vi "Configure Tag Math.vi"(0 "VISA resource name":refnum<visa-resource-name>, 5 "Math Channel (001)":string="001", 7 "Tag Name (\"\")":string, 9 "Tag Number (\"\")":string, 11 "error in (no error)":errorcluster) -> (4 "VISA resource name out":refnum<visa-resource-name>, 6 "Math Channel":string, 15 "error out":errorcluster)   [LabVIEW 2020, in "Yokogawa GX Series.lvlib"]
doc: "Sets the tag of math channel.\n\nCommand: STagMath"
uses:
  <instrlib>/Yokogawa GX Series/Yokogawa GX Series.lvlib
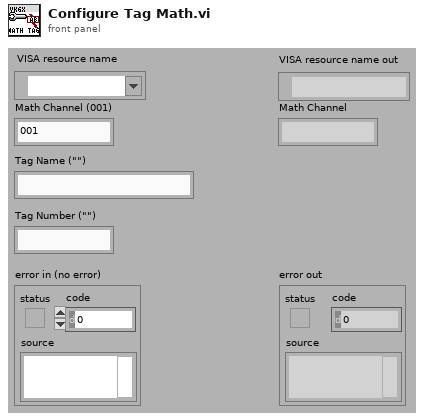
[diagram p1: front panel]
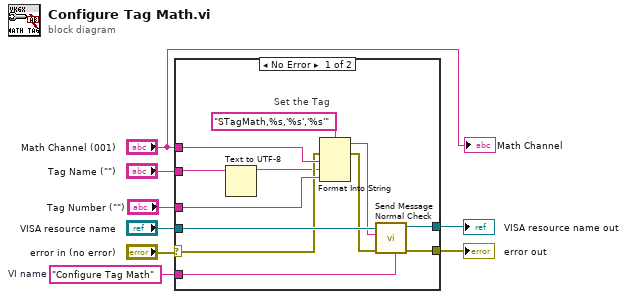
[diagram p0: block diagram]
diagram:
  w6 = "Configure Tag Math"  # VI name
  n1 = case shown="No Error" "error in (no error)" {
    selector: "error in (no error)" -> [w11 w21]
    tunnel: "Tag Name (\"\")" -> [w9 _]
    tunnel: "VISA resource name" -> [w19 w22]
    tunnel: w6 -> [w16 _]
    tunnel: [w15 w22] -> w5
    tunnel: [w14 w21] -> w4
    tunnel: "Tag Number (\"\")" -> [w13 _]
    tunnel: "Math Channel (001)" -> [w12 _]
    frame No Error {
      # "Set the Tag"
      n2 = Text to UTF-8(11:w9) -> (3:w10:string)  [unwired: 2 in, 1 out]
      n3 = Format Into String(format string="STagMath,%s,'%s','%s'", error in=w11, w12, w10, w13) -> (resulting string=w18:string, error out=w17:errorcluster)  [unwired: 1 in]
      n4 = call <instrlib>:"Send Message Normal Check.vi"("Source (\"\")"=w16, "error in (no error)"=w17, "Send Message (\"\")"=w18, "VISA resource name"=w19) -> ("error out"=w14:errorcluster, "VISA resource name out"=w15:refnum<visa-resource-name>)  [unwired: 2 in, 4 out]
    }
    frame Error {
    }
  }
  "error out" <- w4
  "VISA resource name out" <- w5
  "Math Channel" <- "Math Channel (001)"
